vi "TARGET.vi"() -> ()   [LabVIEW 2017]
uses:
  <vilib>/Platform/TimedLoop/XDataNode/timing_clust.ctl
  <vilib>/Platform/TimedLoop/XDataNode/nitl_modes.ctl
  <vilib>/Platform/TimedLoop/XDataNode/wakeup.ctl
  <vilib>/Amulet Technologies/Amulet Display API/Amulet Write Byte.vi
  <vilib>/Amulet Technologies/Amulet Display API/Amulet Write Word.vi
  <vilib>/Amulet Technologies/Amulet Display API/Amulet Write String.vi
  <vilib>/Amulet Technologies/Amulet Display API/Amulet Read Color.vi
  <vilib>/FPGAPlugInAG/cRIO-9067/niLvFpga_Open_cRIO-9067.vi
  <vilib>/rvi/interface/common/dynamic/niFpgaDynamicAddResources.vi
  <vilib>/Utility/error.llb/Error Cluster From Error Code.vi
  <vilib>/rvi/errors/niLvFpgaAdjustHostInterfaceError.vi
  <vilib>/FPGAPlugInAG/Dynamic/niLvFpga_Close_Dynamic.vi
  <vilib>/Platform/TimedLoop/XDataNode/XDataNode.xnode
  <vilib>/rvi/interface/nirviOpenFPGA/nirviOpenFPGA.xnode
  FPGA Bitfiles/Pneumobil_FPGATarget2_MyFPGA_opfJaq9XjZY.lvbitx
  FPGA.vi
  <vilib>/rvi/interface/nirviReadWriteControl/nirviReadWriteControl.xnode
  <vilib>/rvi/interface/nirviCloseFPGA/nirviCloseFPGA.xnode
  <vilib>/Platform/TimedLoop/XDataNode/XDNodeRunTimeDep.lvlib
  <vilib>/rvi/interface/Simulation/niFpgaSimulationCallBeginRW.vi
  NiFpgaLv.dll
  <vilib>/Analysis/NI_AALBase.lvlib
panel:
  out "ResetButtonState":u32
  out "CountsOnReset":u64
  in  "Calc mean":bool
  out "Mean velocity":dbl
  out "Area":dbl
  in  "ECO":bool
  out "Counts":u64
  out "Velocity":dbl
  out "Pressure":dbl
  out "Piston_position":dbl
  out "Pedal_tilt":dbl
  out "Piston_velocity":dbl
  out "Consumption":dbl
  out "Force":dbl
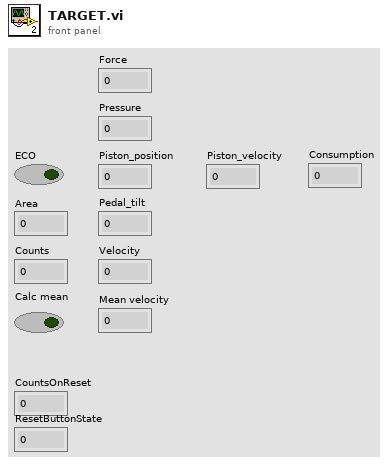
[diagram p1: front panel]
types:
  T1 = typedef "XDNodeRunTimeDep.lvlib/timing_clust.ctl" = cluster{"Expected End [f-1]":u64, "Actual End [f-1]":u64, "Finished Late? [f-1]":bool, "Expected End [i-1]":u64, "Actual End [i-1]":u64, "Finished Late? [i-1]":bool, "Expected Start [i]":u64, "Actual Start [i]":u64, "Expected Start [f]":u64, "Actual Start [f]":u64, "Source Name":string, "Structure Name":string, "Period":i64, "Deadline":i64, "Offset":i64, "Start":i64, "Priority":i32, "Timeout":i32, "Mode":T2, "Wakeup Reason":T3, "Error":errorcluster, "Source Type":string, "Secondary Source Type":string, "Global End Time":u64, "Global Start Time":u64, "Frame Duration":u64, "Iteration Duration":u64, "Assigned CPU":i32, "I/O Scan Engine Mode":u32}
  T2 = typedef "XDNodeRunTimeDep.lvlib/nitl_modes.ctl" = enum32{"No Change", "Process missed periods, maintain original phase", "Discard missed periods, maintain original phase", "Process missed periods, ignore original phase", "Discard missed periods, ignore original phase"}
  T3 = typedef "XDNodeRunTimeDep.lvlib/wakeup.ctl" = enum32{"Normal", "Aborted", "Asynchronous wakeup", "Timing source error", "Timed loop error", "Timeout"}
  T4 = typedef "Amulet VISA Resource Cluster.ctl" = cluster{"VISA resource name":refnum<visa-resource-name>, "Retries":u32, "Host ID":u8, "Amulet ID":u8, "Communication Baud":u32, "Programming Baud":u32}
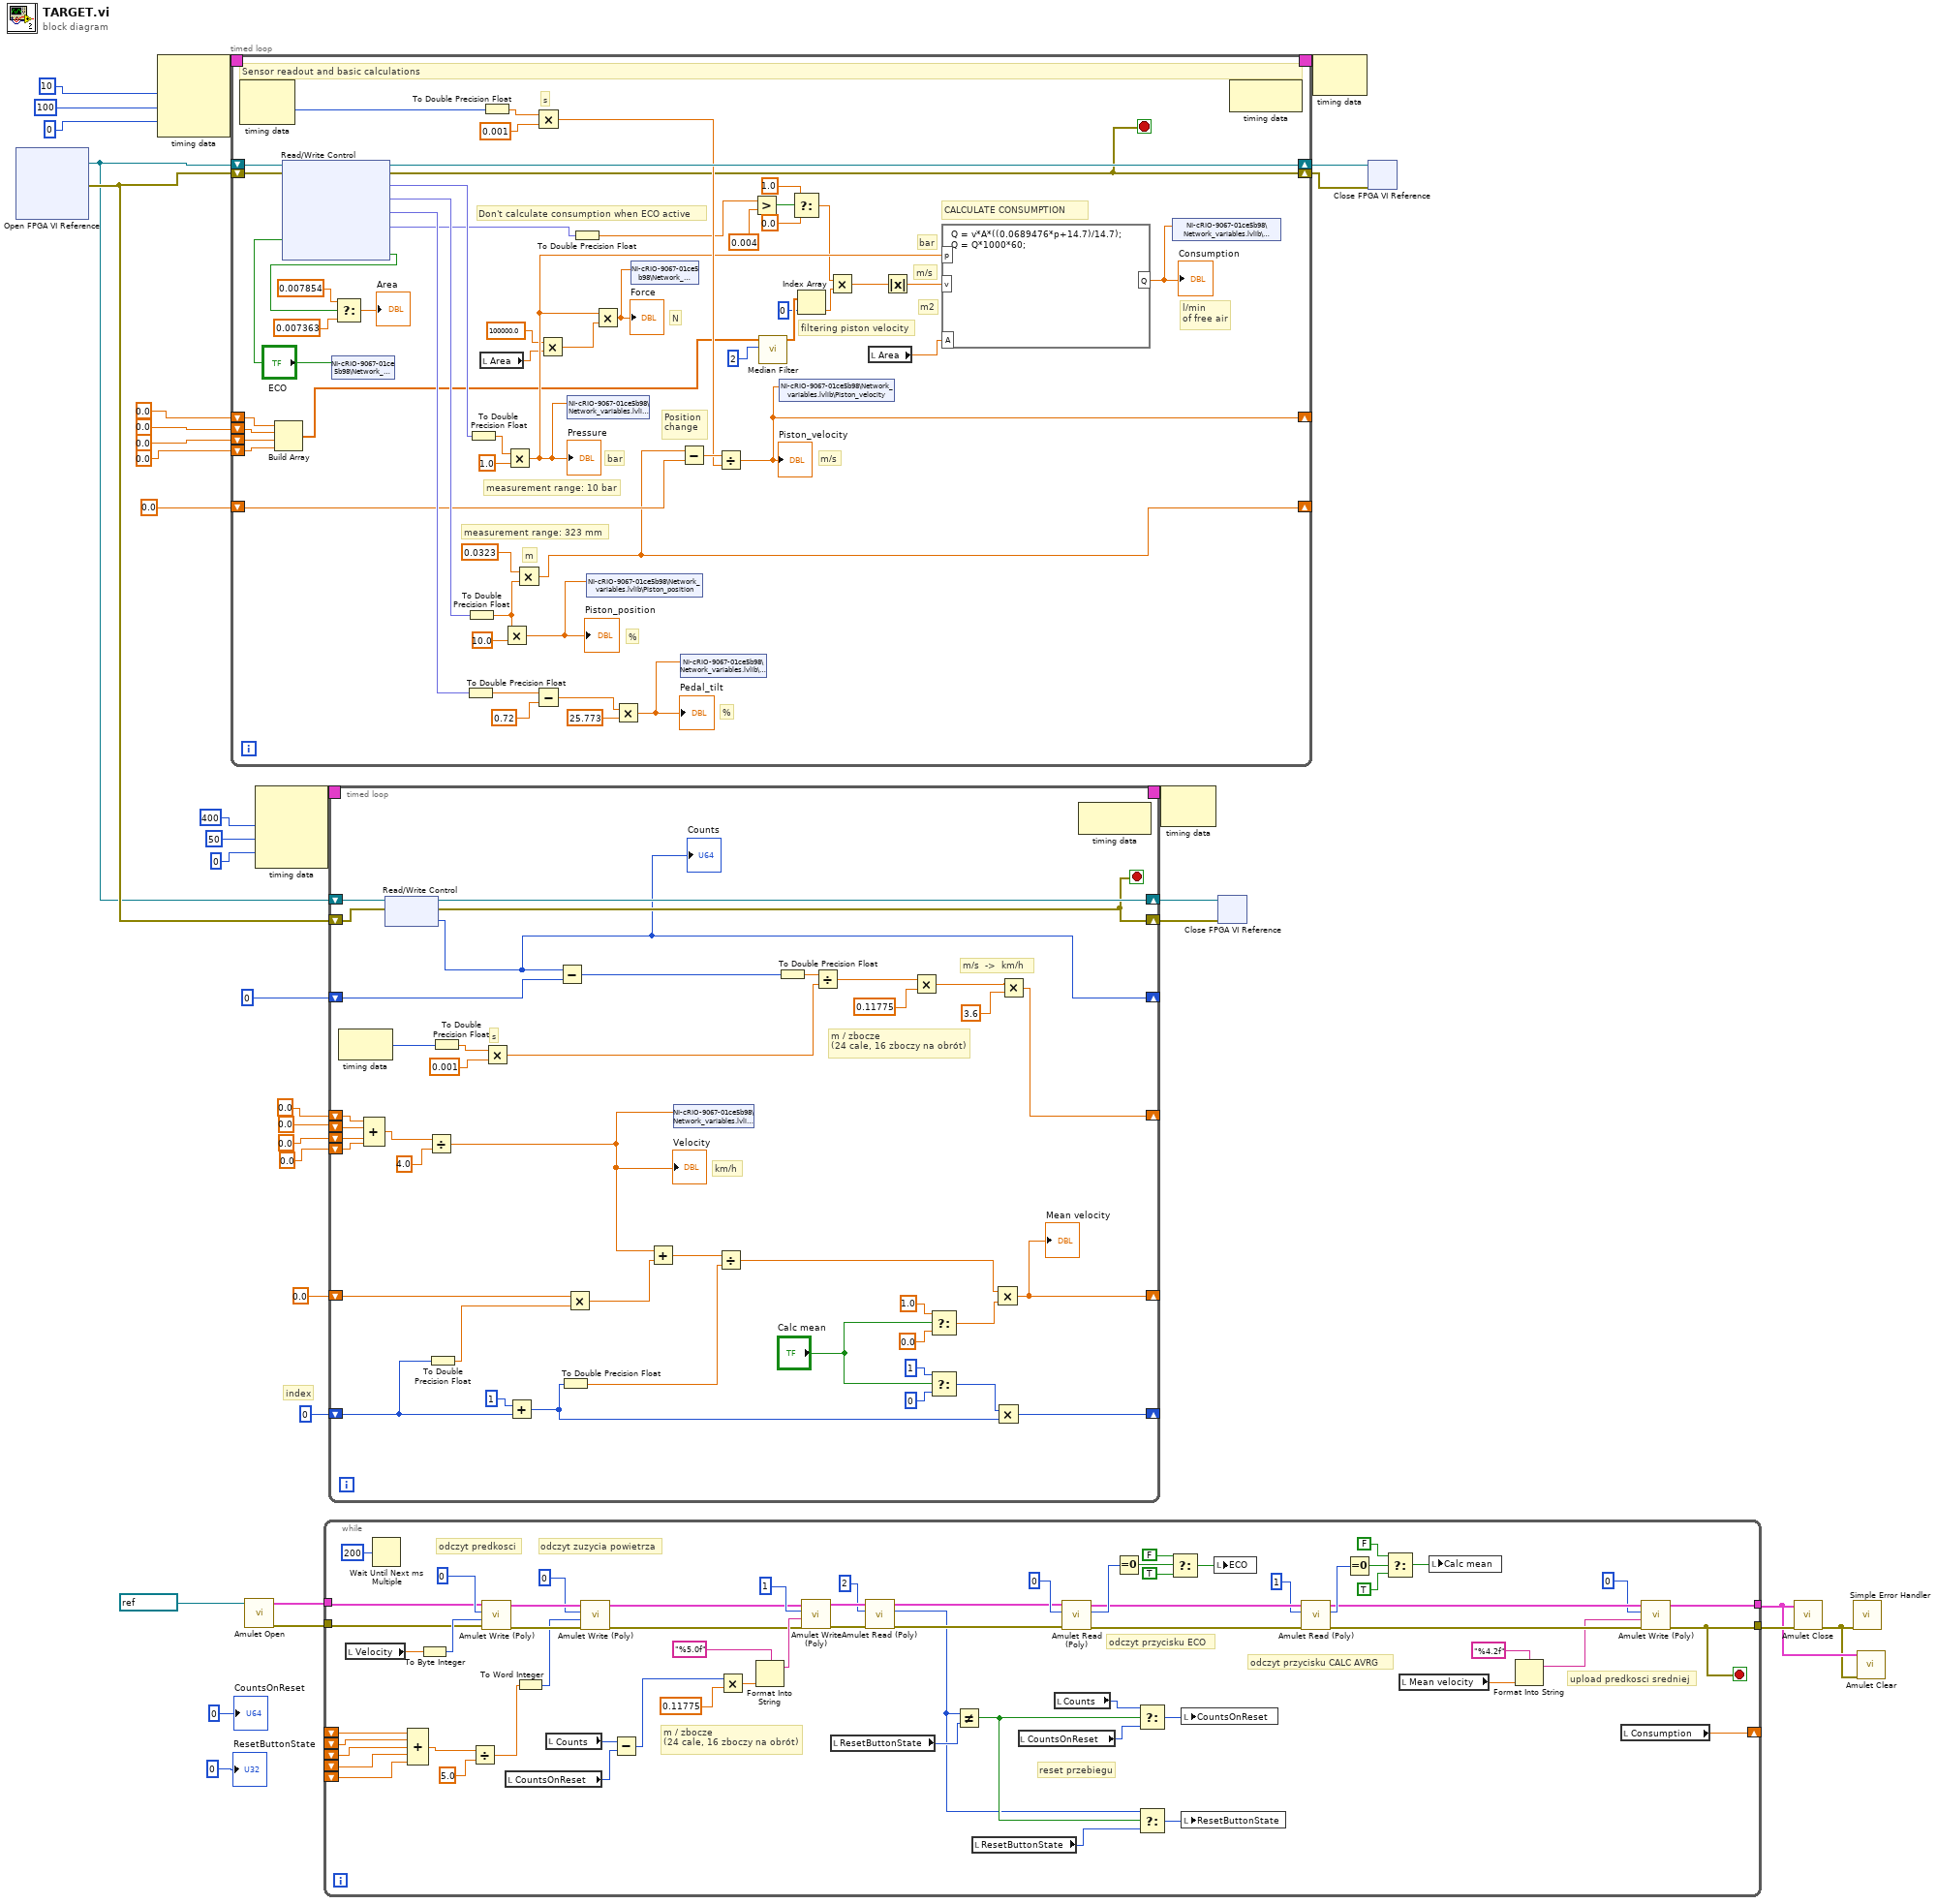
[diagram p0: block diagram]
diagram:
  # "index"
  n1 = xnode "Open FPGA VI Reference"() -> ("FPGA VI Reference Out"=w16:refnum<k20>, "error out"=w17:errorcluster)  [unwired: 2 in]
  n2 = node-c288(i64 10 ("Period"), 100 ("Priority"), i64 0 ("Offset")) -> (w36:T1)  [unwired: 1 in]
  n3 = timed-loop {
    timing: w36 -> [_]
    timing-out: [_] -> w35
    shift-right: [w75] -> w33
    shift-left: w17 -> [w92]
    shift-right: [w90] -> w34
    shift-left: w16 -> [w91]
    shift-right: [w65] -> _
    shift-left: 0.0 -> [w82]
    shift-right: [w38] -> _
    shift-left: 0.0 -> [w59]
    shift-left: 0.0 -> [w58]
    shift-left: 0.0 -> [w52]
    shift-left: 0.0 -> [w51]
    stop <- w75 stop-if-true
    # "filtering piston velocity"
    # "Don't calculate consumption when ECO active"
    # "s"
    # "%"
    # "measurement range: 10 bar"
    # "measurement range: 323 mm"
    # "Position\nchange"
    # "N"
    # "l/min\nof free air"
    # "bar"
    # "m2"
    # "bar"
    # "m/s"
    # "%"
    # "m"
    # "m/s"
    # "CALCULATE CONSUMPTION"
    # "Sensor readout and basic calculations"
    n4 = node-c288() -> (w79:i64)  [unwired: 1 in, 1 out]
    n5 = Build Array(w59, w58, w52, w51) -> (w56:dbl[])
    n6 = xnode "Read/Write Control"("FPGA VI Reference In"=w91, "error in"=w92, "ECO"="ECO") -> ("FPGA VI Reference Out"=w90:refnum<k20>, "error out"=w75:errorcluster, "Pressure"=w89:fxp<+/-,20,5>, "Piston_position"=w88:fxp<+/-,20,5>, "Pedal_tilt"=w87:fxp<+/-,20,5>, "Pressure_regulator"=w50:fxp<+/-,64,44>, "WYSUW"=w46:bool)
    n7 = shared-variable "NI-cRIO-9067-01ce5b98\\Network_variables.lvlib\\ECO"("ECO") -> ()  [unwired: 1 in, 1 out]
    n8 = Select(t=0.007854, s=w46, f=0.007363) -> (s? t:f=→"Area":dbl)
    n9 = To Double Precision Float(number=w87) -> (double precision float=w74:dbl)
    n10 = To Double Precision Float(number=w88) -> (double precision float=w66:dbl)
    n11 = To Double Precision Float(number=w89) -> (double precision float=w86:dbl)
    n12 = local read "Area"() -> (w41:dbl)
    n13 = To Double Precision Float(number=w79) -> (double precision float=w78:dbl)
    n14 = Multiply(x=w66, y=10.0) -> (x*y=w39:dbl)
    "Piston_position" <- w39
    n15 = Multiply(x=w86, y=1.0) -> (x*y=w69:dbl)
    "Pressure" <- w69
    n16 = Multiply(x=0.0323, y=w66) -> (x*y=w65:dbl)
    n17 = Multiply(x=w78, y=0.001 ("x")) -> (x*y=w76:dbl)
    n18 = Subtract(x=w74, y=0.72) -> (x-y=w73:dbl)
    n19 = Multiply(x=100000.0, y=w41) -> (x*y=w40:dbl)
    n20 = shared-variable "NI-cRIO-9067-01ce5b98\\Network_variables.lvlib\\Pressure"(w69) -> ()  [unwired: 1 in, 1 out]
    n21 = To Double Precision Float(number=w50) -> (double precision float=w49:dbl)
    n22 = shared-variable "NI-cRIO-9067-01ce5b98\\Network_variables.lvlib\\Piston_position"(w39) -> ()  [unwired: 1 in, 1 out]
    n23 = Multiply(x=w69, y=w40) -> (x*y=w71:dbl)
    "Force" <- w71
    n24 = Multiply(x=w73, y=25.773) -> (x*y=w68:dbl)
    "Pedal_tilt" <- w68
    n25 = shared-variable "NI-cRIO-9067-01ce5b98\\Network_variables.lvlib\\Force"(w71) -> ()  [unwired: 1 in, 1 out]
    n26 = Subtract(x=w65, y=w82) -> (x-y=w81:dbl)
    n27 = shared-variable "NI-cRIO-9067-01ce5b98\\Network_variables.lvlib\\Pedal_tilt"(w68) -> ()  [unwired: 1 in, 1 out]
    n28 = Divide(x=w81, y=w76) -> (x/y=w38:dbl)
    "Piston_velocity" <- w38
    n29 = Greater?(x=w49, y=0.004) -> (0:w64:bool)
    n30 = call <vilib>:"Median Filter.vi"("left rank"=2, "X"=w56) -> ("Filtered X"=w55:dbl[])  [unwired: 8 in, 1 out]
    n31 = shared-variable "NI-cRIO-9067-01ce5b98\\Network_variables.lvlib\\Piston_velocity"(w38) -> ()  [unwired: 1 in, 1 out]
    n32 = Select(t=1.0, s=w64, f=0.0) -> (s? t:f=w61:dbl)
    n33 = Index Array(array=w55, index=0) -> (element=w53:dbl)
    n34 = Multiply(x=w61, y=w53) -> (x*y=w37:dbl)
    n35 = local read "Area"() -> (w43:dbl)
    n36 = Absolute Value(x=w37) -> (abs(x)=w80:dbl)
    n37 = formula code="Q = v*A*((0.0689476*p+14.7)/14.7);\nQ = Q*1000*60;"("v"=w80, "A"=w43, "p"=w69) -> ("Q"=w70:dbl)
    "Consumption" <- w70
    n38 = shared-variable "NI-cRIO-9067-01ce5b98\\Network_variables.lvlib\\Consumption"(w70) -> ()  [unwired: 1 in, 1 out]
    n39 = node-c288() -> ()  [unwired: 1 in, 1 out]
  }
  n40 = call <vilib>:"Amulet Open.vi"("VISA resource name"=refnum<visa-resource-name> "COM0") -> ("error out"=w21:errorcluster, "Amulet Resource Name"=w22:T4)  [unwired: 9 in]
  n41 = node-c288(i64 400 ("Period"), 50 ("Priority"), i64 0 ("Offset")) -> (w29:T1)  [unwired: 1 in]
  n42 = while {
    tunnel: w22 -> [w148]
    tunnel: w21 -> [w147]
    tunnel: [w132] -> w19
    tunnel: [w133] -> w20
    shift-right: [w127] -> _
    shift-left: _ -> [w124]
    shift-left: _ -> [w123]
    shift-left: _ -> [w122]
    shift-left: _ -> [w121]
    shift-left: _ -> [w120]
    stop <- w133 stop-if-true
    # "odczyt zuzycia powietrza"
    # "odczyt predkosci"
    # "upload predkosci sredniej"
    # "odczyt przycisku CALC AVRG"
    # "odczyt przycisku ECO"
    # "reset przebiegu"
    # "m / zbocze\n(24 cale, 16 zboczy na obrót)"
    n43 = local read "Velocity"() -> (w144:dbl)
    n44 = Wait Until Next ms Multiple(millisecond multiple=u32 200) -> ()  [unwired: 1 out]
    n45 = Compound Arithmetic op=ADD(w124, w123, w122, w121, w120) -> (w125:dbl)
    n46 = To Byte Integer(number=w144) -> (8bit integer=w150:i8)
    n47 = Divide(x=w125, y=5.0) -> (x/y=w119:dbl)
    n48 = call-poly <vilib>:"Amulet Write (Poly).vi"("error in (no error)"=w147, "Byte Value"=w150, "Index"=u8 0, "Amulet Resource Name In"=w148) -> ("error out"=w158:errorcluster, "Amulet Resource Name Out"=w157:T4)  [unwired: 6 in]
    n49 = local read "CountsOnReset"() -> (w105:u64)
    n50 = To Word Integer(number=w119) -> (16bit integer=w155:i16)
    n51 = local read "Counts"() -> (w106:u64)
    n52 = call-poly <vilib>:"Amulet Write (Poly).vi"("error in (no error)"=w158, "Value"=w155, "Index"=u8 0, "Amulet Resource Name In"=w157) -> ("error out"=w114:errorcluster, "Amulet Resource Name Out"=w115:T4)  [unwired: 6 in]
    n53 = Subtract(x=w106, y=w105) -> (x-y=w104:u64)
    n54 = Multiply(x=w104, y=0.11775) -> (x*y=w113:dbl)
    n55 = Format Into String(format string="%5.0f", w113) -> (resulting string=w116:string)  [unwired: 2 in, 1 out]
    n56 = call-poly <vilib>:"Amulet Write (Poly).vi"("error in (no error)"=w114, "Value"=w116, "Index"=u8 1, "Amulet Resource Name In"=w115) -> ("error out"=w111:errorcluster, "Amulet Resource Name Out"=w110:T4)  [unwired: 6 in]
    n57 = local read "ResetButtonState"() -> (w102:u32)
    n58 = call-poly <vilib>:"Amulet Read (Poly).vi"("error in (no error)"=w111, "Index"=u8 2, "Amulet Resource Name In"=w110) -> ("error out"=w108:errorcluster, "Value"=w99:u32, "Amulet Resource Name Out"=w109:T4)  [unwired: 6 in]
    n59 = Not Equal?(x=w99, y=w102) -> (x != y?=w101:bool)
    n60 = local read "ResetButtonState"() -> (w100:u32)
    n61 = local read "CountsOnReset"() -> (w97:u64)
    n62 = local read "Counts"() -> (w96:u64)
    n63 = call-poly <vilib>:"Amulet Read (Poly).vi"("error in (no error)"=w108, "Index"=u8 0, "Amulet Resource Name In"=w109) -> ("error out"=w142:errorcluster, "Value"=w151:u32, "Amulet Resource Name Out"=w143:T4)  [unwired: 6 in]
    n64 = Equal To 0?(x=w151) -> (x = 0?=w152:bool)
    n65 = Select(t=w96, s=w101, f=w97) -> (s? t:f=w103:u64)
    n66 = Select(t=w99, s=w101, f=w100) -> (s? t:f=w98:u32)
    n67 = Select(t=FALSE, s=w152, f=TRUE) -> (s? t:f=w154:bool)
    n68 = local write "CountsOnReset"(w103) -> ()
    n69 = local write "ResetButtonState"(w98) -> ()
    n70 = local write "ECO"(w154) -> ()
    n71 = call-poly <vilib>:"Amulet Read (Poly).vi"("error in (no error)"=w142, "Index"=u8 1, "Amulet Resource Name In"=w143) -> ("error out"=w134:errorcluster, "Value"=w139:u32, "Amulet Resource Name Out"=w135:T4)  [unwired: 6 in]
    n72 = Equal To 0?(x=w139) -> (x = 0?=w140:bool)
    n73 = Select(t=FALSE, s=w140, f=TRUE) -> (s? t:f=w138:bool)
    n74 = local read "Mean velocity"() -> (w130:dbl)
    n75 = local write "Calc mean"(w138) -> ()
    n76 = Format Into String(format string="%4.2f", w130) -> (resulting string=w128:string)  [unwired: 2 in, 1 out]
    n77 = local read "Consumption"() -> (w127:dbl)
    n78 = call-poly <vilib>:"Amulet Write (Poly).vi"("error in (no error)"=w134, "Value"=w128, "Index"=u8 0, "Amulet Resource Name In"=w135) -> ("error out"=w133:errorcluster, "Amulet Resource Name Out"=w132:T4)  [unwired: 6 in]
  }
  n79 = timed-loop {
    timing: w29 -> [_]
    timing-out: [_] -> w28
    shift-right: [w196] -> w24
    shift-left: w16 -> [w198]
    shift-right: [w195] -> w23
    shift-left: w17 -> [w197]
    shift-right: [w187] -> _
    shift-left: u64 0 ("Counts") -> [w186]
    shift-right: [w185] -> _
    shift-left: 0.0 -> [w183]
    shift-left: 0.0 -> [w182]
    shift-left: 0.0 -> [w181]
    shift-left: 0.0 -> [w180]
    shift-right: [w170] -> _
    shift-left: u64 0 -> [w173]
    shift-right: [w161] -> _
    shift-left: 0.0 -> [w177]
    stop <- w195 stop-if-true
    # "m/s  ->  km/h"
    # "m / zbocze\n(24 cale, 16 zboczy na obrót)"
    # "km/h"
    # "s"
    n80 = node-c288() -> (w199:i64)  [unwired: 1 in]
    n81 = Compound Arithmetic op=ADD(w183, w182, w181, w180) -> (w179:dbl)
    n82 = xnode "Read/Write Control"("FPGA VI Reference In"=w198, "error in"=w197) -> ("FPGA VI Reference Out"=w196:refnum<k20>, "error out"=w195:errorcluster, "Counts"=w187:u64)
    "Counts" <- w187
    n83 = Divide(x=w179, y=4.0) -> (x/y=w160:dbl)
    "Velocity" <- w160
    n84 = To Double Precision Float(number=w173) -> (double precision float=w172:dbl)
    n85 = To Double Precision Float(number=w199) -> (double precision float=w201:dbl)
    n86 = Multiply(x=w201, y=0.001 ("x")) -> (x*y=w188:dbl)
    n87 = Add(x=u64 1, y=w173) -> (x+y=w171:u64)
    n88 = Subtract(x=w187, y=w186) -> (x-y=w190:u64)
    n89 = To Double Precision Float(number=w171) -> (double precision float=w174:dbl)
    n90 = Multiply(x=w177, y=w172) -> (x*y=w176:dbl)
    n91 = Add(x=w160, y=w176) -> (x+y=w175:dbl)
    n92 = shared-variable "NI-cRIO-9067-01ce5b98\\Network_variables.lvlib\\Velocity"(w160) -> ()  [unwired: 1 in, 1 out]
    n93 = Divide(x=w175, y=w174) -> (x/y=w169:dbl)
    n94 = To Double Precision Float(number=w190) -> (double precision float=w189:dbl)
    n95 = Divide(x=w189, y=w188) -> (x/y=w191:dbl)
    n96 = Multiply(x=w191, y=0.11775) -> (x*y=w194:dbl)
    n97 = Select(t=1.0, s="Calc mean", f=0.0) -> (s? t:f=w168:dbl)
    n98 = Select(t=u64 1, s="Calc mean", f=u64 0) -> (s? t:f=w162:u64)
    n99 = Multiply(x=w169, y=w168) -> (x*y=w161:dbl)
    "Mean velocity" <- w161
    n100 = Multiply(x=w162, y=w171) -> (x*y=w170:u64)
    n101 = Multiply(x=w194, y=3.6) -> (x*y=w185:dbl)
    n102 = node-c288() -> ()  [unwired: 1 in, 1 out]
  }
  n103 = node-c288(w28) -> ()  [unwired: 1 out]
  n104 = xnode "Close FPGA VI Reference"("FPGA VI Reference In"=w24, "error in"=w23) -> ()  [unwired: 1 out]
  n105 = node-c288(w35) -> ()  [unwired: 1 out]
  n106 = xnode "Close FPGA VI Reference"("FPGA VI Reference In"=w34, "error in"=w33) -> ()  [unwired: 1 out]
  n107 = call <vilib>:"Amulet Close.vi"("error in (no error)"=w20, "Amulet Resource Name In"=w19) -> ("error out"=w18:errorcluster)  [unwired: 9 in]
  n108 = call <vilib>:"Simple Error Handler.vi"("error in (no error)"=w18) -> ()  [unwired: 4 in, 5 out]
  n109 = call <vilib>:"Amulet Clear.vi"("error in (no error)"=w18, "Amulet Resource Name In"=w19) -> ()  [unwired: 8 in, 2 out]
  "CountsOnReset" <- u64 0 ("CountsOnReset")
  "ResetButtonState" <- u32 0 ("ResetButtonState")
